vi "observacao_0MQ.vi"() -> ()   [LabVIEW 2012, in "Shared_160.lvlib"] (continued)
            # "MUDANÇA:\nDesligada chave do\nacompanhamento."
            n3073 = local write "MOUNT"(FALSE ("Led Start/Stop")) -> ()
            n3074 = global write "Global_Telescopio.vi" "STOP ALL"(TRUE ("STOP ALL")) -> ()
          }
        }
        n3075 = case shown="True" "STOP" {
          frame False {
          }
          frame True {
            n3076 = stacked-sequence {
              frame #0 {
                n3077 = call "Stop.vi"() -> ()  [unwired: 1 in, 1 out]
              }
              frame #1 {
                w3999 = 0 ("estado")
                n3078 = local write "statDEC"(w3999) -> ()
                n3079 = local write "statAH"(w3999) -> ()
                n3080 = local write "statCUP"(w3999) -> ()
              }
              frame #2 {
                w4000 = 0 ("estado")
                n3081 = local write "M_AH"(w4000) -> ()
                n3082 = local write "M_DEC"(w4000) -> ()
                n3083 = local write "M_CUP"(w4000) -> ()
                n3084 = local write "M_PROT"(w4000) -> ()
              }
              frame #3 {
                w4001 = FALSE
                n3085 = local write "BtUtilZenith"(w4001) -> ()
                n3086 = local write "BtUtilPark"(w4001) -> ()
                n3087 = local write "FLAT-FIELD"(w4001) -> ()
                n3088 = local write "ECASS"(w4001) -> ()
                n3089 = local write "PROTEÇÃO"(w4001) -> ()
              }
              frame #4 {
                n3090 = case shown="True" "LedPointing" {
                  frame False {
                  }
                  frame True {
                    n3091 = local write "LedPointing"(FALSE ("LedPointing")) -> ()
                    n3092 = global write "Global_Telescopio.vi" "Botão GO = STOP"(TRUE ("Botão GO = STOP")) -> ()
                  }
                }
              }
            }
          }
        }
        n3093 = control-ref of="BtTargetPoint"() -> (w3967:refnum<vi>)
        n3094 = global read "Global_Telescopio.vi" "Centragem Via Aquisicao"() -> (w3974:bool)
        n3095 = property class="Bool"(reference=w3967) -> ("Boolean Text.Text"=w3968:string)  [unwired: 1 in, 2 out]
        n3096 = And(x="Enable Centragem", y=w3974) -> (x .and. y?=w3973:bool)
        n3097 = Or(x="BtOnTatget", y=w3973) -> (x .or. y?=w3970:bool)
        n3098 = local read "FLAT-FIELD"() -> (w3960:bool)
        n3099 = local read "BtUtilZenith"() -> (w3961:bool)
        n3100 = Equal?(x=w3968, y="STOP") -> (x = y?=w3966:bool)
        n3101 = Not(x=w3966) -> (.not. x?=w3965:bool)
        n3102 = And(x=w3965, y=w3970) -> (x .and. y?=w3971:bool)
        n3103 = Or(x=w3961, y=w3960) -> (x .or. y?=w3962:bool)
        n3104 = case shown="True" w3971 {
          frame False {
          }
          frame True {
            n3105 = stacked-sequence {
              seq-local: [w4011 _ _ _ _] -> [_ _ _ _ w4124]
              seq-local: [_ w4025 _ _ _] -> [_ _ _ _ w4125]
              seq-local: [_ _ w4039 _ _] -> [_ _ _ _ w4126]
              seq-local: [_ _ _ w4072 _] -> [_ _ _ _ w4102]
              frame #0 {
                # "Transforma estados lógicos\nnuma string hexadecimal"
                n3106 = local read "Processa Centragem"() -> (w4015:bool)
                n3107 = local read "MOV_IDX_AH"() -> (w4013:bool)
                n3108 = local read "ChkModel"() -> (w4017:bool)
                n3109 = local read "MOV_IDX_DEC"() -> (w4012:bool)
                n3110 = global read "Global_Telescopio.vi" "CalLocal"() -> (w4019:bool)
                n3111 = global read "Global_Telescopio.vi" "CalGlobal"() -> (w4018:bool)
                n3112 = global read "Global_Telescopio.vi" "CoordDia"() -> (w4016:bool)
                n3113 = global read "Global_Telescopio.vi" "ObjCentrado"() -> (w4014:bool)
                n3114 = Build Array(w4019, w4018, w4017, w4016, w4015, w4014, w4013, w4012) -> (w4022:bool[])
                n3115 = Boolean Array To Number(Boolean array=w4022) -> (number=w4021:u32)
                n3116 = Number To Hexadecimal String(1:i16 2 ("width (-)"), 2:w4021) -> (0:w4011:string)
              }
              frame #1 {
                w4026 = "\t"
                # "Reseta Flag do comando oriundo\nda comunicação serial Aquisição"
                n3117 = local read "ChkPointPrecessed"() -> (w4023:bool)
                n3118 = local read "StrPointObjName"() -> (w4029:string)
                "NAME" <- w4029
                n3119 = local read "StrPointObjRA"() -> (w4028:string)
                "RA" <- w4028
                n3120 = local read "StrPointObjDEC"() -> (w4027:string)
                "DEC" <- w4027
                n3121 = case shown="True" w4023 {
                  tunnel: ["2000.000000000" ("Saída") w4033] -> w4024
                  frame False {
                  }
                  frame True {
                    # "20240805"
                    n3122 = call "Calcula epoch.vi"() -> ("epoch"=w4036:dbl)  [unwired: 2 in]
                    n3123 = Number To Fractional String(number=w4036, precision (6)=i16 9) -> (F-format string=w4034:string)  [unwired: 2 in]
                    n3124 = call "Comma_to_Point.vi"("Lat_A"=w4034) -> ("Saída"=w4033:string)
                  }
                }
                n3125 = global write "Global_Telescopio.vi" "Centragem Via Aquisicao"(FALSE ("Centragem Via Aquisicao")) -> ()
                n3126 = local write "Processa Centragem"(TRUE) -> ()
                n3127 = global write "Global_Telescopio.vi" "NAME OBJETO"(w4029) -> ()
                n3128 = global write "Global_Telescopio.vi" "DEC AQUIS"(w4027) -> ()
                n3129 = global write "Global_Telescopio.vi" "RA AQUIS"(w4028) -> ()
                n3130 = Concatenate Strings(w4029, w4026, w4028, w4026, w4027) -> (w4025:string)
                n3131 = global write "Global_Telescopio.vi" "EPOCH AQUIS"(w4024) -> ()
              }
              frame #2 {
                w4037 = "\t"
                w4052 = FALSE ("use system decimal point (T)")
                w4053 = i16 1 ("precision (6)")
                n3132 = global read "Global_Telescopio.vi" "Right Ascention"() -> (w4043:string)
                n3133 = global read "Global_Telescopio.vi" "Calagem DEC"() -> (w4069:dbl)
                n3134 = global read "Global_Telescopio.vi" "Calagem AH"() -> (w4066:dbl)
                n3135 = global read "Global_Telescopio.vi" "Sideral Time"() -> (w4062:dbl)
                n3136 = global read "Global_Telescopio.vi" "Sideral time"() -> (w4040:string)
                n3137 = global read "Global_Telescopio.vi" "Hour Angle"() -> (w4041:string)
                n3138 = global read "Global_Telescopio.vi" "Declination"() -> (w4042:string)
                n3139 = global read "Global_Telescopio.vi" "TargetDEC"() -> (w4057:dbl)
                n3140 = local read "Offset DEC"() -> (w4055:dbl)
                n3141 = global read "Global_Telescopio.vi" "TargetRA"() -> (w4056:dbl)
                n3142 = local read "Offset RA"() -> (w4054:dbl)
                n3143 = global read "Global_Telescopio.vi" "PosDEC"() -> (w4060:dbl)
                n3144 = global read "Global_Telescopio.vi" "PosAH"() -> (w4063:dbl)
                n3145 = local read "UT"() -> (w4038:string)
                n3146 = Subtract(x=w4062, y=w4063) -> (x-y=w4061:dbl)
                n3147 = call "rad_hms.vi"("TRUE=HORA\nFALSE=GRAU"=TRUE ("TRUE=HORA\nFALSE=GRAU"), "Radiano"=w4056) -> ("Hora/Graus Texto Decimal"=w4050:string)  [unwired: 3 in]
                n3148 = call "rad_hms.vi"("TRUE=HORA\nFALSE=GRAU"=FALSE ("TRUE=HORA\nFALSE=GRAU"), "Radiano"=w4057) -> ("Hora/Graus Texto Decimal"=w4049:string)  [unwired: 3 in]
                n3149 = call "rad_hms.vi"("TRUE=HORA\nFALSE=GRAU"=TRUE ("TRUE=HORA\nFALSE=GRAU"), "Radiano"=w4061) -> ("Hora/Graus Texto Decimal"=w4048:string)  [unwired: 3 in]
                n3150 = call "rad_hms.vi"("TRUE=HORA\nFALSE=GRAU"=FALSE ("TRUE=HORA\nFALSE=GRAU"), "Radiano"=w4060) -> ("Hora/Graus Texto Decimal"=w4047:string)  [unwired: 3 in]
                n3151 = call "rad_hms.vi"("TRUE=HORA\nFALSE=GRAU"=TRUE, "Radiano"=w4066) -> ("Hora/Graus Texto Decimal"=w4046:string)  [unwired: 3 in]
                n3152 = call "rad_hms.vi"("TRUE=HORA\nFALSE=GRAU"=FALSE, "Radiano"=w4069) -> ("Hora/Graus Texto Decimal"=w4051:string)  [unwired: 3 in]
                n3153 = Number To Fractional String(use system decimal point (T)=w4052, number=w4055, precision (6)=w4053) -> (F-format string=w4045:string)  [unwired: 1 in]
                n3154 = Number To Fractional String(use system decimal point (T)=w4052, number=w4054, precision (6)=w4053) -> (F-format string=w4044:string)  [unwired: 1 in]
                n3155 = Concatenate Strings(w4050, w4037, w4049, w4037, w4048, w4037, w4047, w4037, w4046, w4037, w4051, w4037, w4045, w4037, w4044, w4037, w4043, w4037, w4042, w4037, w4041, w4037, w4040, w4037, w4038) -> (w4039:string)
              }
              frame #3 {
                w4071 = TRUE
                w4070 = FALSE
                w4073 = "\t"
                # "MUDANÇA 30-03-2024: Inseridos no LOG  os valores de coordenadas de \ninteresse para um levantamento de erros de apontamento do telescópio."
                n3156 = global read "Global_Telescopio.vi" "PointingModel DEC"() -> (w4095:dbl)
                n3157 = global read "Global_Telescopio.vi" "PointingModel RA"() -> (w4096:dbl)
                n3158 = global read "Global_Telescopio.vi" "Precessed  DEC"() -> (w4097:dbl)
                n3159 = global read "Global_Telescopio.vi" "Calagem DEC"() -> (w4099:dbl)
                n3160 = global read "Global_Telescopio.vi" "Precessed RA"() -> (w4098:dbl)
                n3161 = global read "Global_Telescopio.vi" "CalDEC Local"() -> (w4100:dbl)
                n3162 = global read "Global_Telescopio.vi" "Calagem AH"() -> (w4101:dbl)
                n3163 = global read "Global_Telescopio.vi" "CalAH Local"() -> (w4094:dbl)
                n3164 = global read "Global_Telescopio.vi" "Sideral Time"() -> (w4087:dbl)
                n3165 = global read "Global_Telescopio.vi" "PosDEC"() -> (w4088:dbl)
                n3166 = global read "Global_Telescopio.vi" "PosAH"() -> (w4086:dbl)
                n3167 = Subtract(x=w4096, y=w4094) -> (x-y=w4093:dbl)
                n3168 = Add(x=w4095, y=w4100) -> (x+y=w4091:dbl)
                n3169 = Subtract(x=w4087, y=w4086) -> (x-y=w4089:dbl)
                n3170 = Subtract(x=w4093, y=w4101) -> (x-y=w4092:dbl)
                n3171 = Add(x=w4091, y=w4099) -> (x+y=w4090:dbl)
                n3172 = call "rad_hms.vi"("TRUE=HORA\nFALSE=GRAU"=w4071, "Radiano"=w4098) -> ("Hora/Graus Texto Decimal"=w4074:string)  [unwired: 3 in]
                n3173 = call "rad_hms.vi"("TRUE=HORA\nFALSE=GRAU"=w4070, "Radiano"=w4097) -> ("Hora/Graus Texto Decimal"=w4075:string)  [unwired: 3 in]
                n3174 = call "rad_hms.vi"("TRUE=HORA\nFALSE=GRAU"=w4071, "Radiano"=w4096) -> ("Hora/Graus Texto Decimal"=w4076:string)  [unwired: 3 in]
                n3175 = call "rad_hms.vi"("TRUE=HORA\nFALSE=GRAU"=w4070, "Radiano"=w4095) -> ("Hora/Graus Texto Decimal"=w4077:string)  [unwired: 3 in]
                n3176 = call "rad_hms.vi"("TRUE=HORA\nFALSE=GRAU"=w4071, "Radiano"=w4093) -> ("Hora/Graus Texto Decimal"=w4078:string)  [unwired: 3 in]
                n3177 = call "rad_hms.vi"("TRUE=HORA\nFALSE=GRAU"=w4070, "Radiano"=w4091) -> ("Hora/Graus Texto Decimal"=w4079:string)  [unwired: 3 in]
                n3178 = call "rad_hms.vi"("TRUE=HORA\nFALSE=GRAU"=w4071, "Radiano"=w4092) -> ("Hora/Graus Texto Decimal"=w4080:string)  [unwired: 3 in]
                n3179 = call "rad_hms.vi"("TRUE=HORA\nFALSE=GRAU"=w4070, "Radiano"=w4090) -> ("Hora/Graus Texto Decimal"=w4081:string)  [unwired: 3 in]
                n3180 = call "rad_hms.vi"("TRUE=HORA\nFALSE=GRAU"=w4071, "Radiano"=w4089) -> ("Hora/Graus Texto Decimal"=w4082:string)  [unwired: 3 in]
                n3181 = call "rad_hms.vi"("TRUE=HORA\nFALSE=GRAU"=w4070, "Radiano"=w4088) -> ("Hora/Graus Texto Decimal"=w4083:string)  [unwired: 3 in]
                n3182 = call "rad_hms.vi"("TRUE=HORA\nFALSE=GRAU"=w4071, "Radiano"=w4087) -> ("Hora/Graus Texto Decimal"=w4084:string)  [unwired: 3 in]
                n3183 = call "rad_hms.vi"("TRUE=HORA\nFALSE=GRAU"=w4071, "Radiano"=w4086) -> ("Hora/Graus Texto Decimal"=w4085:string)  [unwired: 3 in]
                n3184 = Concatenate Strings(w4074, w4073, w4075, w4073, w4076, w4073, w4077, w4073, w4078, w4073, w4079, w4073, w4080, w4073, w4081, w4073, w4082, w4073, w4083, w4073, w4084, w4073, w4085) -> (w4072:string)
              }
              frame #4 {
                w4123 = "\t"
                # "MUDANÇA 30-03-2024: Apenas afeta o arquivo de LOG se e somente se o nome do objeto apontado contiver o caracter @. Neste caso o LOG é feito num arquivo separado cujo nome é formado pela data (mesma do arquivo log regular) acrescido do caracter @. O conteúdo deste novo LOG apenas difere do regular pela inclusão no início de cada registro do timestamp, do nome do objeto apontado (sem o @) e dos valores de RA e DEC, em radianos, de todas as etapas do processo de apontamento."
                # "Coordenadas da precessão, modelagem erros, calagem e lidas do encoder"
                # "Condições atmosféricas"
                # "Dados de catálogo do Objeto"
                # "Tempo e posição do telescópio"
                # "Estados das variáveis de processos"
                n3185 = global read "Global_Telescopio.vi" "NAME OBJETO"() -> (w4117:string)
                n3186 = Get Date/Time In Seconds() -> (seconds since 1Jan1904=w4109:timestamp)
                n3187 = local read "AtmosferaStr"() -> (w4121:string)
                n3188 = global read "Global_Telescopio.vi" "Data Arq LOG"() -> (w4135:string)
                n3189 = Format Date/Time String(time format string (%c)="%c%3u" ("SOMENTE DIRETORIO"), seconds (now)=w4109) -> (date/time string=w4103:string)  [unwired: 1 in]
                n3190 = Match Pattern(string=w4117, regular expression="@" ("SOMENTE DIRETORIO")) -> (before substring=w4111:string, match substring=w4114:string, after substring=w4112:string, offset past match=w4108:i32)  [unwired: 1 in]
                n3191 = Greater Or Equal To 0?(x=w4108) -> (x >= 0?=w4107:bool)
                n3192 = Concatenate Strings("C:\\TCS\\LOG\\AP_" ("SOMENTE DIRETORIO"), w4135, w4114, ".TXT" ("SOMENTE DIRETORIO")) -> (w4113:string)
                n3193 = Concatenate Strings(w4111, w4112) -> (w4104:string)
                n3194 = Concatenate Strings(w4126, w4123, w4125, w4123, w4121, w4123, w4124, "\r\n") -> (w4106:string)
                n3195 = case shown="True" w4107 {
                  tunnel: w4106 -> [w4137 w4139]
                  tunnel: [w4137 w4143] -> w4105
                  tunnel: w4104 -> [_ w4141]
                  tunnel: w4103 -> [_ w4142]
                  tunnel: w4102 -> [_ w4140]
                  frame False {
                  }
                  frame True {
                    w4138 = "\t"
                    n3196 = Concatenate Strings(w4142, w4138, w4141, w4138, w4140, w4138, w4139) -> (w4143:string)
                  }
                }
                n3197 = String To Path(string=w4113) -> (path=w4134:path)
                n3198 = call <vilib>:"Open_Create_Replace File.vi"("function (open:0)"=T9."open or create", "file path"=w4134) -> ("error out"=w4131:errorcluster, "refnum"=w4132:refnum<file>)  [unwired: 6 in, 2 out]
                n3199 = Set File Position(refnum=w4132, from (0:start)=enum16{"start", "end", "current"}."end" ("pos mode (0:2)"), error in=w4131) -> (refnum out=w4120:refnum<file>, error out=w4119:errorcluster)  [unwired: 1 in]
                n3200 = Write to Binary File(file (use dialog)=w4120, data=w4105, error in=w4119, 5:FALSE ("prepend array or string size? (T)")) -> (refnum out=w4128:refnum<file>, error out=w4129:errorcluster)  [unwired: 2 in, 1 out]
                n3201 = Close File(refnum=w4128, error in=w4129) -> (error out=w4127:errorcluster)  [unwired: 1 out]
                n3202 = call <vilib>:"Simple Error Handler.vi"("error in (no error)"=w4127) -> ()  [unwired: 4 in, 5 out]
              }
            }
          }
        }
        n3203 = case shown="False" w3962 {
          frame False {
            w3980 = u16 3 items=["Alarme", "Atencao", "Erro", "Ocupado", "Protecao", "Embreagem", "Tracking", "Var. Track", "Rápido", "Ligeiro", "Médio", "Lento", "Em movimento", ""] ("NomeStatus")
            n3204 = call "Bit Status AH.vi"("NomeStatus"=w3980) -> ("StatBit"=w3979:bool)
            n3205 = case shown="True" "MOUNT" {
              tunnel: w3979 -> [w3982 w3991]
              frame False {
                n3206 = local read "LED MOUNT"() -> (w3983:bool)
                n3207 = Not(x=w3982) -> (.not. x?=w3985:bool)
                n3208 = And(x=w3985, y=w3983) -> (x .and. y?=w3984:bool)
                n3209 = case shown="True" w3984 {
                  frame False {
                  }
                  frame True {
                    w3987 = FALSE
                    w3988 = u16 1 items=["ZERO", "AH", "DEC", "TUBO", "CUP"] ("Controlador")
                    n3210 = call "Monta Comando.vi"("Comando"="DESLIGAR", "Dispositivo"="SIDERAL" ("Comando"), "Controlador"=w3988) -> ()  [unwired: 4 in, 3 out]
                    n3211 = local write "LED MOUNT"(w3987) -> ()
                    n3212 = global write "Global_Telescopio.vi" "ObjCentrado"(w3987) -> ()
                    n3213 = property on="Calagem" class="Bool"("Disabled"=u8 2) -> ()  [unwired: 2 in, 2 out]
                  }
                }
              }
              frame True {
                n3214 = local read "LED MOUNT"() -> (w3992:bool)
                n3215 = Or(x=w3991, y=w3992) -> (x .or. y?=w3993:bool)
                n3216 = case shown="True" w3993 {
                  frame False {
                    w3994 = u16 1 items=["ZERO", "AH", "DEC", "TUBO", "CUP"] ("Controlador")
                    n3217 = call "Monta Comando.vi"("Comando"="LIGAR", "Dispositivo"="SIDERAL" ("Comando"), "Controlador"=w3994) -> ()  [unwired: 4 in, 3 out]
                    "LED MOUNT" <- TRUE
                  }
                  frame True {
                  }
                }
              }
            }
          }
          frame True {
            n3218 = local write "LED MOUNT"(FALSE) -> ()
          }
        }
      }
      frame #4 {
        # "Abre Imagens"
        # "ABAS DE IMAGENS"
        n3219 = case shown="\"All Sky\"" "Tab Control" {
          frame "Image 1", Default {
            n3220 = disable-structure shown="Disabled" {
              frame Disabled {
                # "Imagem oriunda do\nconector BNC 1"
                n3221 = global read "Global_Telescopio.vi" "Tempo Atulização Cam 0"() -> (w4152:i16)
                n3222 = call "timepulse_Cam_0.vi"("de quantos segundos"=w4152) -> ("PULSO"=w4155:bool)  [unwired: 2 in]
                n3223 = Or(x="IMAGE 5", y=w4155) -> (x .or. y?=w4154:bool)
                n3224 = case shown="True" w4154 {
                  frame False {
                  }
                  frame True {
                    n3225 = call "AngeloRTV_Snap.vi"("PortNo"=u16 0) -> ("depth"=w4161:u8, "color table"=w4159:u32[], "rect"=w4162:T13, "flattened image data"=w4160:u8[])  [unwired: 2 in, 1 out]
                    n3226 = call <vilib>:"Draw Flattened Pixmap(6_1).vi"("bit depth(8)"=w4161, "rect"=w4162, "flattened pixmap data"=w4160, "color table"=w4159) -> ("new picture"=→"Image":picture)  [unwired: 5 in]
                    n3227 = call "Acerta_moldura.vi"("fator"=i16 1, "input cluster"=w4162) -> ("Draw Area Size"=w4156:cluster{"Width":u32, "Height":u32})  [unwired: 3 in]
                    n3228 = property on="Image" class="Pict"("Draw Area Size"=w4156) -> ()  [unwired: 2 in, 2 out]
                  }
                }
              }
              frame Enabled {
              }
            }
          }
          frame "All Sky" {
            n3229 = global read "Global_Telescopio.vi" "Tempo Atulização All Sky"() -> (w4164:i16)
            n3230 = call "timepulse_Cam_4.vi"("de quantos segundos"=w4164) -> ("PULSO"=w4165:bool)  [unwired: 2 in]
            n3231 = Or(x="IMAGE 2", y=w4165) -> (x .or. y?=w4166:bool)
            n3232 = case shown="True" w4166 {
              frame False {
              }
              frame True {
                n3233 = stacked-sequence {
                  frame #0 {
                    # "Deixado Propositalmente caso queira colocar uma camera no local do ALL SKY"
                    n3234 = case shown="True" "Case Constant\n(See Context Help) 16" {
                      frame False {
                      }
                      frame True {
                        # "Coloca a moldura na\nImagem"
                        # "Imagen da Cam Setada"
                        n3235 = call "AngeloRTV_Snap.vi"("PortNo"=u16 2) -> ("depth"=w4174:u8, "color table"=w4172:u32[], "rect"=w4175:T13, "flattened image data"=w4173:u8[])  [unwired: 2 in, 1 out]
                        n3236 = call "Acerta_moldura.vi"("fator"=i16 1, "input cluster"=w4175) -> ("Draw Area Size"=w4170:cluster{"Width":u32, "Height":u32})  [unwired: 3 in]
                        "Draw Area 2" <- w4170
                        n3237 = call <vilib>:"Draw Flattened Pixmap(6_1).vi"("bit depth(8)"=w4174, "rect"=w4175, "flattened pixmap data"=w4173, "color table"=w4172) -> ("new picture"=→"Image 2":picture)  [unwired: 5 in]
                        n3238 = property on="Image 2" class="Pict"("Draw Area Size"=w4170) -> ()  [unwired: 2 in, 2 out]
                      }
                    }
                  }
                  frame #1 {
                    # "Fora do ar\n12/02/2009"
                    n3239 = case shown="True" "Case Constant\n(See Context Help) 17" {
                      frame False {
                      }
                      frame True {
                        n3240 = stacked-sequence {
                          seq-local: [w4181 _] -> [_ w4190]
                          frame #0 {
                            n3241 = String To Path(string="C:\\TCSPD_TRABALHO\\IMAGE_TEMP.JPG") -> (path=w4185:path)
                            n3242 = call "URL Get HTTP Document.vi"("follow redirects (T)"="follow redirects (T)", "file path (NAP)"=w4185, "http URL"="http://200.131.64.207/allsky/imagens/allsky_opd.jpg") -> ("error out"=w4180:errorcluster, "file path out"=w4181:path, "header"=→"header":string)  [unwired: 1 in, 5 out]
                            "error out 2" <- w4180
                            n3243 = Unbundle By Name(w4180) -> ("status"=w4179:bool)
                            n3244 = case shown="True" w4179 {
                              frame False {
                              }
                              frame True {
                                n3245 = One Button Dialog(message="Erro durante a aquisição da Imagem do All Sky do site:\n\nhttp://200.131.64.207/allsky/imagens/allsky_opd.jpg") -> ()  [unwired: 1 in, 1 out]
                              }
                            }
                          }
                          frame #1 {
                            (unwired) path "\\\\200.131.64.207/allsky/imagens/allsky_opd.jpg\\" ("path to JPEG file")
                            (unwired) "\\Nasa - Earth From Outer Space.jpg" ("caminho final")
                            # "Isto não está sendo mais usado porémmantive se caso\nseja necessário a manipulação de arquivos com imagem"
                            # "fator de \nredução \nSomente\ninteiros até 6"
                            # "Sem nome de\narquivo ele abre\ncaixa de Diálogo"
                            # "Coloca a moldura na\nImagem"
                            # "Imagen da Cam Setada"
                            n3246 = String To Path(string="/root/Desktop/Simulador/Nasa - Earth From Outer Space.jpg" ("caminho final")) -> ()  [unwired: 1 out]
                            n3247 = call "Read JPEG File(6_1).vi"("path to JPEG file"=w4190) -> ("error out"=w4199:errorcluster, "flattened image data"=w4196:u8[], "rect"=w4195:T13, "colorTable"=w4198:u32[], "depth"=w4197:u8)  [unwired: 5 in, 1 out]
                            "error out 3" <- w4199
                            n3248 = call "Fator_Reducao.vi"("rect"=w4195, "flattened image in"=w4196, "Fator Tamanho"=i16 4) -> ("flattened image out"=w4194:u8[], "area figura x e y"=w4189:cluster{"X Resolution":i32, "Y Resolution":i32})  [unwired: 2 out]
                            n3249 = call "Webcam Flat to Picture.vi"("color table"=w4198, "depth 24/8"=w4197, "error in"=w4199, "rect in"=w4195, "flat image in"=w4194) -> ("error out"=→"error out 4":errorcluster, "picture"=w4188:picture)  [unwired: 2 in, 2 out]
                            n3250 = local write "Draw Area 2"(w4189) -> ()
                            n3251 = property on="Image 2" class="Pict"("Draw Area Size"=w4189) -> ()  [unwired: 2 in, 2 out]
                            n3252 = local write "Image 2"(w4188) -> ()
                            n3253 = call "Cria_path_local.vi"("caminho final"="\\allsky_opd.jpg") -> ()  [unwired: 3 in, 2 out]
                          }
                        }
                      }
                    }
                  }
                }
              }
            }
          }
          frame "Finder" {
            # "Imagem oriunda do\nconector BNC 4"
            n3254 = global read "Global_Telescopio.vi" "Tempo Atulização Cam 3"() -> (w4200:i16)
            n3255 = call "timepulse_Cam_3.vi"("de quantos segundos"=w4200) -> ("PULSO"=w4201:bool)  [unwired: 2 in]
            n3256 = Or(x="IMAGE 4", y=w4201) -> (x .or. y?=w4203:bool)
            n3257 = case shown="True" w4203 {
              frame False {
              }
              frame True {
                n3258 = stacked-sequence {
                  frame #0 {
                    n3259 = call "AngeloRTV_Snap.vi"("PortNo"=u16 3) -> ("depth"=w4209:u8, "color table"=w4207:u32[], "rect"=w4210:T13, "flattened image data"=w4208:u8[])  [unwired: 2 in, 1 out]
                    n3260 = call "Acerta_moldura.vi"("fator"=i16 1, "input cluster"=w4210) -> ("Draw Area Size"=w4204:cluster{"Width":u32, "Height":u32})  [unwired: 3 in]
                    "Draw Area 4" <- w4204
                    n3261 = call <vilib>:"Draw Flattened Pixmap(6_1).vi"("bit depth(8)"=w4209, "rect"=w4210, "flattened pixmap data"=w4208, "color table"=w4207) -> ("new picture"=→"Image 4":picture)  [unwired: 5 in]
                    n3262 = property on="Image 4" class="Pict"("Draw Area Size"=w4204) -> ()  [unwired: 2 in, 2 out]
                  }
                  frame #1 {
                    n3263 = case shown="True" "Case Constant\n(See Context Help) 18" {
                      frame False {
                      }
                      frame True {
                        # "Isto não está sendo mais usado porémmantive se caso\nseja necessário a manipulação de arquivos com imagem"
                        # "fator de \nredução \nSomente\ninteiros até 6"
                        # "Sem nome de\narquivo ele abre\ncaixa de Diálogo"
                        # "Coloca a moldura na\nImagem"
                        # "Imagen da Cam Setada"
                        n3264 = call "Cria_path_local.vi"("caminho final"="\\Nasa - Earth From Outer Space.jpg") -> ("Saida Path inteiro"=w4215:path)  [unwired: 3 in, 1 out]
                        n3265 = call "Read JPEG File(6_1).vi"("path to JPEG file"=w4215) -> ("error out"=w4224:errorcluster, "flattened image data"=w4221:u8[], "rect"=w4220:T13, "colorTable"=w4223:u32[], "depth"=w4222:u8)  [unwired: 5 in, 1 out]
                        n3266 = String To Path(string="/root/Desktop/Simulador/Nasa - Earth From Outer Space.jpg" ("caminho final")) -> ()  [unwired: 1 out]
                        n3267 = call "Fator_Reducao.vi"("rect"=w4220, "flattened image in"=w4221, "Fator Tamanho"=i16 1) -> ("flattened image out"=w4219:u8[], "area figura x e y"=w4213:cluster{"X Resolution":i32, "Y Resolution":i32})  [unwired: 2 out]
                        n3268 = local write "Draw Area 4"(w4213) -> ()
                        n3269 = property on="Image 4" class="Pict"("Draw Area Size"=w4213) -> ()  [unwired: 2 in, 2 out]
                        n3270 = call "Webcam Flat to Picture.vi"("color table"=w4223, "depth 24/8"=w4222, "error in"=w4224, "rect in"=w4220, "flat image in"=w4219) -> ("picture"=w4214:picture)  [unwired: 2 in, 3 out]
                        n3271 = local write "Image 4"(w4214) -> ()
                      }
                    }
                  }
                }
              }
            }
          }
          frame "Telescope" {
            # "Imagem oriunda do\nconector BNC 2"
            n3272 = global read "Global_Telescopio.vi" "Tempo Atulização Cam 1"() -> (w4225:i16)
            n3273 = call "timepulse_Cam_1.vi"("de quantos segundos"=w4225) -> ("PULSO"=w4226:bool)  [unwired: 2 in]
            n3274 = Or(x="IMAGE 3", y=w4226) -> (x .or. y?=w4227:bool)
            n3275 = case shown="True" w4227 {
              frame False {
              }
              frame True {
                n3276 = case shown="True" "Case Constant\n(See Context Help) 19" {
                  frame False {
                  }
                  frame True {
                    n3277 = call "AngeloRTV_Snap.vi"("PortNo"=u16 1) -> ("depth"=w4235:u8, "color table"=w4233:u32[], "rect"=w4236:T13, "flattened image data"=w4234:u8[])  [unwired: 2 in, 1 out]
                    n3278 = call <vilib>:"Draw Flattened Pixmap(6_1).vi"("bit depth(8)"=w4235, "rect"=w4236, "flattened pixmap data"=w4234, "color table"=w4233) -> ("new picture"=→"Image 3":picture)  [unwired: 5 in]
                    n3279 = call "Acerta_moldura.vi"("fator"=i16 1, "input cluster"=w4236) -> ("Draw Area Size"=w4230:cluster{"Width":u32, "Height":u32})  [unwired: 3 in]
                    "Draw Area 3" <- w4230
                    n3280 = property on="Image 3" class="Pict"("Draw Area Size"=w4230) -> ()  [unwired: 2 in, 2 out]
                  }
                }
              }
            }
          }
          frame "Image 3" {
            # "Imagem oriunda do\nconector BNC 3"
            n3281 = global read "Global_Telescopio.vi" "Tempo Atulização Cam 2"() -> (w4238:i16)
            n3282 = call "timepulse_Cam_2.vi"("de quantos segundos"=w4238) -> ("PULSO"=w4239:bool)  [unwired: 2 in]
            n3283 = Or(x="IMAGE 6", y=w4239) -> (x .or. y?=w4241:bool)
            n3284 = case shown="True" w4241 {
              frame False {
              }
              frame True {
                n3285 = call "AngeloRTV_Snap.vi"("PortNo"=u16 2) -> ("depth"=w4247:u8, "color table"=w4245:u32[], "rect"=w4248:T13, "flattened image data"=w4246:u8[])  [unwired: 2 in, 1 out]
                n3286 = call "Acerta_moldura.vi"("fator"=i16 1, "input cluster"=w4248) -> ("Draw Area Size"=w4242:cluster{"Width":u32, "Height":u32})  [unwired: 3 in]
                n3287 = call <vilib>:"Draw Flattened Pixmap(6_1).vi"("bit depth(8)"=w4247, "rect"=w4248, "flattened pixmap data"=w4246, "color table"=w4245) -> ("new picture"=→"Image 3a":picture)  [unwired: 5 in]
                n3288 = property on="Image 3a" class="Pict"("Draw Area Size"=w4242) -> ()  [unwired: 2 in, 2 out]
              }
            }
          }
          frame "Test Only" {
          }
        }
        n3289 = global read "Global_Telescopio.vi" "Caminho camera"() -> (w4149:string)
        n3290 = global read "Global_Telescopio.vi" "stop"() -> (w4150:bool)
        n3291 = call "Greatek.vi"("error in (no error)"="error in (no error)", "Boolean"=w4150, "name or relative path"=w4149, ".NET Refnum in"="PictureBox") -> ("error out"=→"error out 5":errorcluster)  [unwired: 7 in]
      }
      frame #5 {
        w4265 = u16 3 items=["Alarme", "Atencao", "Erro", "Ocupado", "TBD", "LCB", "Trapeira", "Paravento", "DomoRap", "DomoCW", "DomoCCW", "TBD", "Em movimento", "TBD"] ("NomeStatus")
        # "ZeroMQ"
        # "JANELA DE STATUS"
        n3292 = local read "RA on Target"() -> (w4261:bool)
        n3293 = local read "DEC on Target"() -> (w4260:bool)
        n3294 = local read "Led Chave Dome"() -> (w4257:bool)
        n3295 = local read "Dome on Target"() -> (w4259:bool)
        n3296 = local read "LED GUIDER"() -> (w4256:bool)
        n3297 = local read "MOUNT"() -> (w4258:bool)
        n3298 = local read "Mount Gross Movement"() -> (w4255:bool)
        n3299 = local read "Mount Fine Movement"() -> (w4254:bool)
        n3300 = local read "ObjCentrado"() -> (w4253:bool)
        n3301 = local read "LED VAR TRACKING"() -> (w4252:bool)
        n3302 = local read "LedShutter"() -> (w4251:bool)
        n3303 = local read "StatDome"() -> (w4250:string)
        n3304 = local read "ChkDomeEnable"() -> (w4276:bool)
        n3305 = global write "Global_Telescopio.vi" "PUB StatDome"(w4250) -> ()
        n3306 = global write "Global_Telescopio.vi" "PUB RA on Target"(w4261) -> ()
        n3307 = global write "Global_Telescopio.vi" "PUB DEC on Target"(w4260) -> ()
        n3308 = global write "Global_Telescopio.vi" "PUB Dome"(w4257) -> ()
        n3309 = global write "Global_Telescopio.vi" "PUB Dome on Target"(w4259) -> ()
        n3310 = global write "Global_Telescopio.vi" "PUB GUIDER"(w4256) -> ()
        n3311 = global write "Global_Telescopio.vi" "PUB MOUNT"(w4258) -> ()
        n3312 = global write "Global_Telescopio.vi" "PUB Mount Gross Movement"(w4255) -> ()
        n3313 = global write "Global_Telescopio.vi" "PUB Mount Fine Movement"(w4254) -> ()
        n3314 = global write "Global_Telescopio.vi" "PUB ObjCentrado"(w4253) -> ()
        n3315 = global write "Global_Telescopio.vi" "PUB VAR TRACKING"(w4252) -> ()
        n3316 = global write "Global_Telescopio.vi" "PUB SHUTTER"(w4251) -> ()
        n3317 = local read "Flag Stop"() -> (w4271:bool)
        n3318 = case shown="True" w4276 {
          tunnel: [TRUE ("AUX LAMPADA") w4430] -> w4275
          frame False {
          }
          frame True {
            w4436 = u16 3 items=["Alarme", "Atencao", "Erro", "Ocupado", "TBD", "LCB", "Trapeira", "Paravento", "DomoRap", "DomoCW", "DomoCCW", "TBD", "Em movimento", "TBD"] ("NomeStatus")
            n3319 = local read "Dome on Target"() -> (w4433:bool)
            n3320 = local read "statCUP"() -> (w4435:i32)
            n3321 = call "Bit Status CUP.vi"("NomeStatus"=w4436) -> ("StatBit"=w4432:bool)
            n3322 = Equal To 0?(x=w4435) -> (x = 0?=w4434:bool)
            n3323 = Not(x=w4432) -> (.not. x?=w4431:bool)
            n3324 = Compound Arithmetic op=AND(w4434, w4433, w4431) -> (w4430:bool)
          }
        }
        n3325 = case shown="True" w4271 {
          tunnel: [FALSE w4423] -> w4270
          frame False {
          }
          frame True {
            w4427 = u16 3 items=["Alarme", "Atencao", "Erro", "Ocupado", "TBD", "LCB", "Trapeira", "Paravento", "DomoRap", "DomoCW", "DomoCCW", "TBD", "Em movimento", "TBD"] ("NomeStatus")
            n3326 = local read "statCUP"() -> (w4426:i32)
            n3327 = call "Bit Status CUP.vi"("NomeStatus"=w4427) -> ("StatBit"=w4428:bool)
            n3328 = Equal To 0?(x=w4426) -> (x = 0?=w4425:bool)
            n3329 = Not(x=w4428) -> (.not. x?=w4424:bool)
            n3330 = Compound Arithmetic op=AND(w4425, w4424) -> (w4423:bool)
          }
        }
        n3331 = local read "Flag de erro p/ apagar lampada"() -> (w4266:bool)
        n3332 = local read "Apontou"() -> (w4283:bool)
        n3333 = local read "BtUtilZenith"() -> (w4291:bool)
        n3334 = local read "BtUtilPark"() -> (w4290:bool)
        n3335 = local read "BtUtilZenith"() -> (w4289:bool)
        n3336 = local read "ECASS"() -> (w4288:bool)
        n3337 = local read "FLAT-FIELD"() -> (w4287:bool)
        n3338 = call "Bit Status CUP.vi"("NomeStatus"=w4265) -> ("StatBit"=w4264:bool)
        n3339 = local read "DEC on Target"() -> (w4277:bool)
        n3340 = local read "RA on Target"() -> (w4278:bool)
        n3341 = Compound Arithmetic op=OR(w4283, w4291, w4290, w4289, w4288, w4287) -> (w4284:bool)
        n3342 = And(x=w4284, y="AUX ABA") -> (x .and. y?=w4286:bool)
        n3343 = Not(x=w4264) -> (.not. x?=w4263:bool)
        n3344 = case shown="True" w4286 {
          selector: w4286 -> [_ w4448]
          frame False {
          }
          frame True {
            # "Liga a câmera de monitoramento"
            # "Ligar a lâmpada pra a câmera"
            n3345 = Not(x=w4448) -> (.not. x?=w4447:bool)
            n3346 = local write "AUX ABA"(w4447) -> ()
            n3347 = local write "Apontou"(w4447) -> ()
            n3348 = local write "AUX LAMPADA"(TRUE ("AUX LAMPADA")) -> ()
            n3349 = local write "Tab Control"(T1."Image 1" ("Tab Control")) -> ()
          }
        }
        n3350 = case shown="False" w4284 {
          selector: w4284 -> [w4444 _]
          frame False {
            n3351 = Not(x=w4444) -> (.not. x?=w4445:bool)
            n3352 = local write "AUX ABA"(w4445) -> ()
          }
          frame True {
          }
        }
        n3353 = Compound Arithmetic op=AND(w4266, w4263) -> (w4262:bool)
        n3354 = Compound Arithmetic op=AND(w4278, w4277, w4275) -> (w4274:bool)
        n3355 = And(x=w4274, y="AUX LAMPADA") -> (x .and. y?=w4272:bool)
        n3356 = Or(x=w4272, y=w4270) -> (x .or. y?=w4267:bool)
        n3357 = Or(x=w4267, y=w4262) -> (x .or. y?=w4268:bool)
        n3358 = Not(x=w4278) -> (.not. x?=w4279:bool)
        n3359 = Not(x=w4277) -> (.not. x?=w4281:bool)
        n3360 = Not(x=w4275) -> (.not. x?=w4280:bool)
        n3361 = case shown="True" w4268 {
          selector: w4268 -> [_ w4441]
          frame False {
          }
          frame True {
            w4438 = u16 4 items=["ZERO", "AH", "DEC", "TUBO", "CUP"] ("Controlador")
            n3362 = Not(x=w4441) -> (.not. x?=w4437:bool)
            n3363 = local write "AUX LAMPADA"(w4437) -> ()
            n3364 = local write "Flag Stop"(w4437) -> ()
            n3365 = local write "Flag de erro p/ apagar lampada"(w4437) -> ()
            n3366 = local write "Tab Control"(T1."Test Only" ("Tab Control")) -> ()
            n3367 = call "Monta Comando.vi"("Comando"="DESLIGAR", "Dispositivo"="LAMP_CAM", "Controlador"=w4438) -> ()  [unwired: 4 in, 3 out]
          }
        }
        n3368 = Compound Arithmetic op=OR(w4279, w4281, w4280) -> (w4282:bool)
        n3369 = case shown="True" w4282 {
          selector: w4282 -> [_ w4443]
          frame False {
          }
          frame True {
            n3370 = local write "AUX LAMPADA"(w4443) -> ()
          }
        }
        n3371 = global read "Global_Telescopio.vi" "Enable ventilador"() -> (w4269:bool)
        n3372 = Tick Count (ms)() -> (millisecond timer value=w4294:u32)
        n3373 = case shown="True" w4269 {
          frame False {
          }
          frame True {
            w4300 = u16 3 items=["Alarme", "Atencao", "Erro", "Ocupado", "TBD", "LCB", "Trapeira", "Paravento", "DomoRap", "DomoCW", "DomoCCW", "TBD", "Em movimento", "TBD"] ("NomeStatus")
            n3374 = global read "Global_Telescopio.vi" "Hora vent inicial"() -> (w4297:string)
            n3375 = global read "Global_Telescopio.vi" "Hora vent final"() -> (w4296:string)
            n3376 = call "Bit Status TUBO.vi"("NomeStatus"=w4300) -> ("StatBit"=w4299:bool)
            n3377 = call "Comp-HorarioSeg.vi"("Lower limit"=w4297, "Upper limit"=w4296) -> ("In Range?"=w4295:bool)
            n3378 = Not(x=w4299) -> (.not. x?=w4298:bool)
            n3379 = case shown="\"ligar\"" "xxz" {
              tunnel: [w4303 w4327 w4352 w4356 w4369 w4375 w4388] -> w4301
              tunnel: w4295 -> [_ _ w4351 _ w4371 _ w4389]
              tunnel: w4298 -> [w4304 w4328 _ w4355 w4370 w4374 _]
              frame "erro_ligar" {
                n3380 = case shown="True" w4304 {
                  tunnel: ["erro_ligar" w4306] -> w4303
                  frame False {
                  }
                  frame True {
                    w4315 = u16 3 items=["ZERO", "AH", "DEC", "TUBO", "CUP"] ("Controlador")
                    # "super erro"
                    n3381 = call "Monta Comando.vi"("Comando"="LIGAR", "Dispositivo"="VENTILADOR", "Controlador"=w4315) -> ("Resposta"=w4318:string)  [unwired: 4 in, 2 out]
                    n3382 = String Subset(string=w4318, length (rest)=3 ("length (rest)")) -> (substring=w4312:string)  [unwired: 1 in]
                    n3383 = Equal?(x=w4312, y="ACK") -> (x = y?=w4308:bool)
                    n3384 = case shown="False" w4308 {
                      tunnel: [w4319 FALSE] -> w4309
                      tunnel: "erro_ligar" -> [w4320 _]
                      tunnel: [w4320 "espera_desligar"] -> w4307
                      frame False {
                        n3385 = Increment(x="erro lig") -> (x+1=w4321:i32)
                        n3386 = local write "erro lig"(w4321) -> ()
                        n3387 = Greater Or Equal?(x=w4321, y=3) -> (x >= y?=w4319:bool)
                        n3388 = case shown="True" w4319 {
                          frame False {
                          }
                          frame True {
                            w4324 = "Erro de acionamento do ventilador do tubo" ("SYSTEM MESSAGES")
                            n3389 = call "Monta_Mensagem.vi"("Mensagem"=w4324) -> ()  [unwired: 2 in]
                            n3390 = call "Salva_systems_messages.vi"("Mensagem"=w4324) -> ()  [unwired: 5 in]
                          }
                        }
                      }
                      frame True {
                      }
                    }
                    n3391 = Select(t="espera_desligar", s=w4309, f=w4307) -> (s? t:f=w4306:string)
                  }
                }
              }
              frame "erro_desligar" {
                n3392 = case shown="True" w4328 {
                  tunnel: ["erro_desligar" w4330] -> w4327
                  frame False {
                  }
                  frame True {
                    w4340 = u16 3 items=["ZERO", "AH", "DEC", "TUBO", "CUP"] ("Controlador")
                    # "super erro"
                    n3393 = call "Monta Comando.vi"("Comando"="DESLIGAR", "Dispositivo"="VENTILADOR", "Controlador"=w4340) -> ("Resposta"=w4338:string)  [unwired: 4 in, 2 out]
                    n3394 = String Subset(string=w4338, length (rest)=3 ("length (rest)")) -> (substring=w4336:string)  [unwired: 1 in]
                    n3395 = Equal?(x=w4336, y="ACK") -> (x = y?=w4335:bool)
                    n3396 = case shown="False" w4335 {
                      tunnel: [w4343 FALSE] -> w4334
                      tunnel: "erro_desligar" -> [w4344 _]
                      tunnel: [w4344 "aguardando _ligar"] -> w4332
                      frame False {
                        n3397 = Increment(x="erro des") -> (x+1=w4346:i32)
                        n3398 = local write "erro des"(w4346) -> ()
                        n3399 = Greater Or Equal?(x=w4346, y=3) -> (x >= y?=w4343:bool)
                        n3400 = case shown="True" w4343 {
                          frame False {
                          }
                          frame True {
                            w4348 = "Erro de acionamento do ventilador do tubo" ("SYSTEM MESSAGES")
                            n3401 = call "Monta_Mensagem.vi"("Mensagem"=w4348) -> ()  [unwired: 2 in]
                            n3402 = call "Salva_systems_messages.vi"("Mensagem"=w4348) -> ()  [unwired: 5 in]
                          }
                        }
                      }
                      frame True {
                      }
                    }
                    n3403 = Select(t="aguardando _ligar", s=w4334, f=w4332) -> (s? t:f=w4330:string)
                  }
                }
              }
              frame "inicio", Default {
                n3404 = Select(t="ligar", s=w4351, f="desligar") -> (s? t:f=w4352:string)
              }
              frame "ligar" {
                n3405 = case shown="True" w4355 {
                  tunnel: ["ligar" w4359] -> w4356
                  frame False {
                  }
                  frame True {
                    w4366 = u16 3 items=["ZERO", "AH", "DEC", "TUBO", "CUP"] ("Controlador")
                    n3406 = call "Monta Comando.vi"("Comando"="LIGAR", "Dispositivo"="VENTILADOR", "Controlador"=w4366) -> ("Resposta"=w4364:string)  [unwired: 4 in, 2 out]
                    n3407 = String Subset(string=w4364, length (rest)=3 ("length (rest)")) -> (substring=w4362:string)  [unwired: 1 in]
                    n3408 = Equal?(x=w4362, y="ACK") -> (x = y?=w4358:bool)
                    n3409 = Select(t="espera_desligar", s=w4358, f="erro_ligar") -> (s? t:f=w4359:string)
                  }
                }
              }
              frame "espera_desligar" {
                n3410 = case shown="False" w4371 {
                  tunnel: w4370 -> [_ _]
                  tunnel: ["desligar" "espera_desligar"] -> w4369
                  frame False {
                    # "Já ligou mas saiu da faixa e deve desligar"
                  }
                  frame True {
                    # "Já ligou mas está na faixa"
                  }
                }
              }
              frame "desligar" {
                n3411 = case shown="True" w4374 {
                  tunnel: ["desligar" w4377] -> w4375
                  frame False {
                  }
                  frame True {
                    w4385 = u16 3 items=["ZERO", "AH", "DEC", "TUBO", "CUP"] ("Controlador")
                    n3412 = call "Monta Comando.vi"("Comando"="DESLIGAR", "Dispositivo"="VENTILADOR", "Controlador"=w4385) -> ("Resposta"=w4383:string)  [unwired: 4 in, 2 out]
                    n3413 = String Subset(string=w4383, length (rest)=3 ("length (rest)")) -> (substring=w4381:string)  [unwired: 1 in]
                    n3414 = Equal?(x=w4381, y="ACK") -> (x = y?=w4380:bool)
                    n3415 = Select(t="aguardando _ligar", s=w4380, f="erro_desligar") -> (s? t:f=w4377:string)
                  }
                }
              }
              frame "aguardando _ligar" {
                n3416 = case shown="True" w4389 {
                  tunnel: ["aguardando _ligar" "ligar"] -> w4388
                  frame False {
                  }
                  frame True {
                  }
                }
              }
            }
            n3417 = local write "xxz"(w4301) -> ()
          }
        }
        n3418 = stacked-sequence {
          frame #0 {
            n3419 = Get Date/Time String(want seconds? (F)=TRUE ("Boolean")) -> (time string=w4394:string)  [unwired: 2 in, 1 out]
            n3420 = In Range and Coerce(upper limit="16:00:01", x=w4394, lower limit="15:59:59" ("upper limit")) -> (In Range?=w4393:bool)  [unwired: 1 out]
            n3421 = In Range and Coerce(upper limit="17:45:01", x=w4394, lower limit="17:44:59" ("upper limit")) -> (In Range?=w4392:bool)  [unwired: 1 out]
            n3422 = case shown="True" w4392 {
              selector: w4392 -> [_ w4400]
              frame False {
              }
              frame True {
                "Flag desligar" <- w4400
              }
            }
            n3423 = case shown="True" w4393 {
              selector: w4393 -> [_ w4401]
              frame False {
              }
              frame True {
                "Flag ligar" <- w4401
              }
            }
          }
          frame #1 {
            n3424 = local read "Flag ligar"() -> (w4403:bool)
            n3425 = local read "Flag desligar"() -> (w4402:bool)
            n3426 = Or(x=w4403, y=w4402) -> (x .or. y?=w4404:bool)
            n3427 = case shown="True" w4404 {
              tunnel: w4403 -> [_ w4405]
              tunnel: w4402 -> [_ w4407]
              frame False {
              }
              frame True {
                w4411 = u16 3 items=["Alarme", "Atencao", "Erro", "Ocupado", "TBD", "LCB", "Trapeira", "Paravento", "DomoRap", "DomoCW", "DomoCCW", "TBD", "Em movimento", "TBD"] ("NomeStatus")
                n3428 = call "Bit Status TUBO.vi"("NomeStatus"=w4411) -> ("StatBit"=w4410:bool)
                n3429 = Not(x=w4410) -> (.not. x?=w4406:bool)
                n3430 = And(x=w4406, y=w4407) -> (x .and. y?=w4408:bool)
                n3431 = And(x=w4405, y=w4406) -> (x .and. y?=w4409:bool)
                n3432 = case shown="True" w4409 {
                  selector: w4409 -> [_ w4421]
                  frame False {
                  }
                  frame True {
                    w4419 = u16 3 items=["ZERO", "AH", "DEC", "TUBO", "CUP"] ("Controlador")
                    n3433 = Not(x=w4421) -> (.not. x?=w4420:bool)
                    n3434 = local write "Flag ligar"(w4420) -> ()
                    n3435 = call "Monta Comando.vi"("Comando"="LIGAR", "Dispositivo"="VENTILADOR", "Controlador"=w4419) -> ()  [unwired: 4 in, 3 out]
                  }
                }
                n3436 = case shown="True" w4408 {
                  selector: w4408 -> [_ w4416]
                  frame False {
                  }
                  frame True {
                    w4412 = u16 3 items=["ZERO", "AH", "DEC", "TUBO", "CUP"] ("Controlador")
                    n3437 = Not(x=w4416) -> (.not. x?=w4415:bool)
                    n3438 = local write "Flag desligar"(w4415) -> ()
                    n3439 = call "Monta Comando.vi"("Comando"="DESLIGAR", "Dispositivo"="VENTILADOR", "Controlador"=w4412) -> ()  [unwired: 4 in, 3 out]
                  }
                }
              }
            }
          }
        }
        n3440 = Subtract(x=w4294, y=w4293) -> (x-y=→"dt":u32)
      }
    }
    n3441 = Wait Until Next ms Multiple(millisecond multiple=u32 100) -> ()  [unwired: 1 out]
    n3442 = global read "Global_Telescopio.vi" "stop"() -> (w69:bool)
    n3443 = Or(x=w69, y="sair") -> (x .or. y?=w70:bool)
  }
  n3444 = flat-sequence {
    tunnel: w1 -> [_]
    frame #0 {
      # "Comando EXIT\nP/ O VI QBRIDGE"
      # "Libera as filas do focalizador"
      n3445 = global read "Global_Telescopio.vi" "queueSUB"() -> (w4453:refnum<queue>)
      n3446 = global read "Global_Telescopio.vi" "queuePUSH"() -> (w4452:refnum<queue>)
      n3447 = Enqueue Element(queue=w4452, element="AbortBridge") -> (queue out=w4451:refnum<queue>)  [unwired: 2 in, 2 out]
      n3448 = Release Queue(queue=w4453) -> ()  [unwired: 2 in, 3 out]
      n3449 = Release Queue(queue=w4451) -> ()  [unwired: 2 in, 3 out]
    }
  }
  n3450 = case shown="True" FALSE {
    tunnel: w1 -> [_ w4454]
    frame False {
    }
    frame True {
      n3451 = Quit LabVIEW(quit? (T)=w4454) -> ()
    }
  }
